vi "Vertical Insert-Right.vi"(6 "depth":dbl, 8 "error in":errorcluster, 9 "Speed":dbl=10.0, 11 "Location":string="Base") -> (0 "error out":errorcluster, 3 "Location Out":string="Base")   [LabVIEW 2013]
uses:
  ROS/Code/Console/Servers/ServerSubs/(nist) Arm Globals.vi
panel:
  out "R:Effort at start":dbl[](array[numeric])=[-0.416, -0.52, 1.12, -3.856, -0.084, -0.176, 0.14]
  out "Goal Z":dbl
  out "R:Effort":dbl[](array[numeric])=[-0.416, -0.52, 1.12, -3.856, -0.084, -0.176, 0.14]
  in  "XYZOAT":T1
  in  "MaxAngle":dbl=40.0
  in  "deg/cycle":dbl=2.0
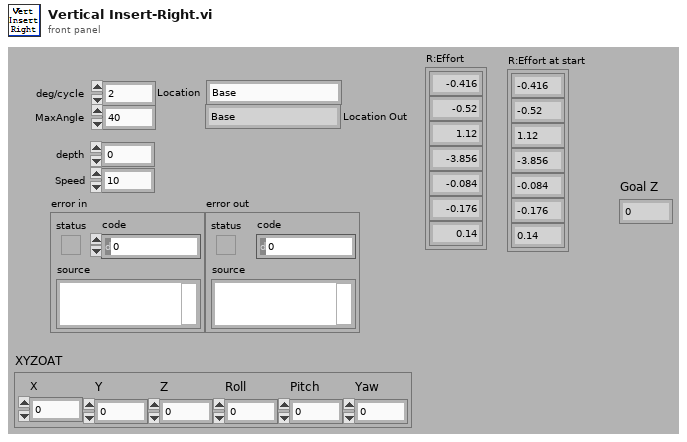
[diagram p1: front panel]
types:
  T1 = cluster{"X":dbl, "Y":dbl, "Z":dbl, "Roll":dbl, "Pitch":dbl, "Yaw":dbl}
  T2 = cluster{"X":dbl, "Y":dbl, "Z":dbl, "O":dbl, "A":dbl, "T":dbl}
  T3 = typedef "NI_Matrix.lvlib/RealMatrix.ctl" = dbl[][]
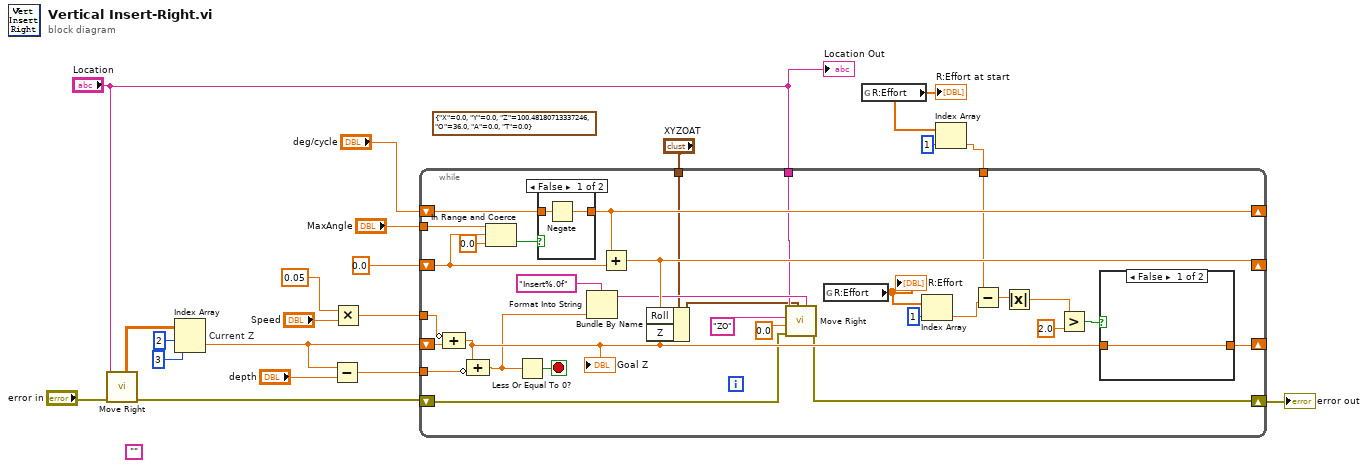
[diagram p0: block diagram]
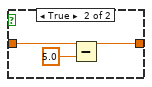
[diagram p2: hidden frame]
diagram:
  (unwired) T2 {"X"=0.0, "Y"=0.0, "Z"=100.48180713337246, "O"=36.0, "A"=0.0, "T"=0.0} ("Goal Axes")
  (unwired) ""
  n1 = call "Move Right.vi"("error in"="error in", "Location"="Location") -> ("error out"=w3:errorcluster, "Current"=w4:T3)  [unwired: 5 in, 3 out]
  n2 = Index Array "Current Z"(array=w4, index (row)=2, index (col)=3) -> (element=w10:dbl)
  n3 = Subtract(x=w10, y="depth") -> (x-y=w9:dbl)
  n4 = Multiply(x=0.05 ("y"), y="Speed") -> (x*y=w18:dbl)
  n5 = global read "(nist) Arm Globals.vi" "R:Effort"() -> (w6:dbl[])
  "R:Effort at start" <- w6
  n6 = Index Array(array=w6, index=1) -> (element=w5:dbl)
  n7 = while {
    tunnel: w9 -> [w51]
    shift-right: [w33] -> _
    shift-left: w10 -> [w50]
    tunnel: w18 -> [w49]
    shift-right: [w43] -> _
    shift-left: "deg/cycle" -> [w47]
    tunnel: "MaxAngle" -> [w45]
    shift-right: [w42] -> _
    shift-left: 0.0 -> [w44]
    shift-right: [w22] -> w15
    shift-left: w3 -> [w23]
    tunnel: "Location" -> [w26]
    tunnel: "XYZOAT" -> [w32]
    tunnel: w5 -> [w29]
    stop <- w41 stop-if-true
    n8 = Compound Arithmetic op=ADD(invert w49, w50) -> (w34:dbl)
    "Goal Z" <- w34
    n9 = Compound Arithmetic op=ADD(w34, invert w51) -> (w31:dbl)
    n10 = In Range and Coerce(upper limit=w45, x=w44, lower limit=0.0) -> (In Range?=w48:bool)  [unwired: 1 out]
    n11 = Less Or Equal To 0?(x=w31) -> (x <= 0?=w41:bool)
    n12 = case shown="False" w48 {
      tunnel: w47 -> [w57 w58]
      tunnel: [w56 w58] -> w43
      frame False {
        n13 = Negate(x=w57) -> (-x=w56:dbl)
      }
      frame True {
      }
    }
    n14 = Format Into String(format string="Insert%.0f", w31) -> (resulting string=w39:string)  [unwired: 2 in, 1 out]
    n15 = Add(x=w43, y=w44) -> (x+y=w42:dbl)
    n16 = Bundle By Name(cluster=w32, "Roll"=w42, "Z"=w34) -> (w25:T1)
    n17 = call "Move Right.vi"("Label"=w39, "Goal"=w25, "error in"=w23, "Speed"=0.0 ("Speed (mm/s)"), "Mask"="ZO", "Location"=w26) -> ("error out"=w22:errorcluster)  [unwired: 1 in, 4 out]
    n18 = global read "(nist) Arm Globals.vi" "R:Effort"() -> (w38:dbl[])
    "R:Effort" <- w38
    n19 = Index Array(array=w38, index=1) -> (element=w30:dbl)
    n20 = Subtract(x=w29, y=w30) -> (x-y=w28:dbl)
    n21 = Absolute Value(x=w28) -> (abs(x)=w27:dbl)
    n22 = Greater?(x=w27, y=2.0) -> (0:w35:bool)
    n23 = case shown="False" w35 {
      tunnel: w34 -> [w52 w55]
      tunnel: [w52 w54] -> w33
      frame False {
      }
      frame True {
        n24 = Subtract(x=w55, y=5.0) -> (x-y=w54:dbl)
      }
    }
  }
  "error out" <- w15
  "Location Out" <- "Location"
